vi "Read captureSpectImage.vi"(8 "error in (no error)":errorcluster, 11 "captureSpectImage in":refnum<class "captureSpectImage.lvclass">) -> (0 "error out":errorcluster, 2 "command_captureSpectImage":T1={"integrationTime"=0.0, "imageType"="                                                                                                                                                                                                                                                                ", "lamp"="                                                                                                                                                                                                                                                                "}, 3 "captureSpectImage out":refnum<class "captureSpectImage.lvclass">)   [LabVIEW 2016, in "Commands.lvlib" / "captureSpectImage.lvclass"]
uses:
  captureSpectImage.lvclass
  ts_sallv_sedspectrometer/DataTypes/command_captureSpectImage.ctl
  captureSpectImage.lvclass/captureSpectImage.ctl
  ts_sallv_sedspectrometer/SALLV_sedSpectrometer.lvlib
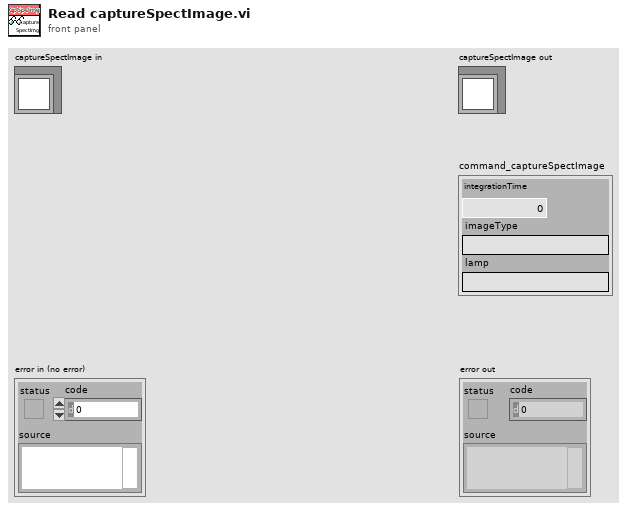
[diagram p1: front panel]
types:
  T1 = typedef "SALLV_sedSpectrometer.lvlib/command_captureSpectImage.ctl" = cluster{"integrationTime":sgl, "imageType":string, "lamp":string}
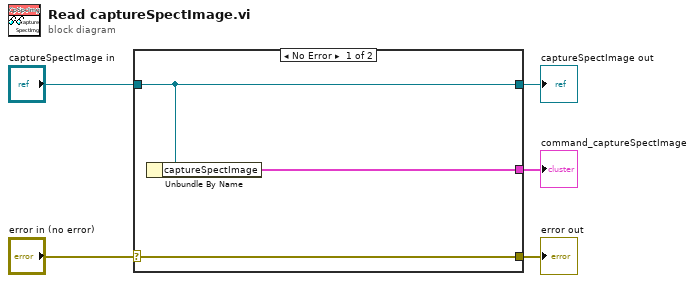
[diagram p0: block diagram]
diagram:
  n1 = case shown="No Error" "error in (no error)" {
    selector: "error in (no error)" -> [w8 w9]
    tunnel: [w8 w9] -> w4
    tunnel: [w7 w10] -> w2
    tunnel: "captureSpectImage in" -> [w7 w10]
    tunnel: [w6 _] -> w1
    frame No Error {
      n2 = Unbundle By Name(w7) -> ("captureSpectImage"=w6:T1)
    }
    frame Error {
    }
  }
  "error out" <- w4
  "captureSpectImage out" <- w2
  "command_captureSpectImage" <- w1
